vi "Read Single Measurement (Voltage).vi"(0 "VISA resource name":refnum<visa-resource-name>, 5 "Maximum Time (10000 ms)":i32=10000, 11 "error in (no error)":errorcluster) -> (4 "VISA resource name out":refnum<visa-resource-name>, 6 "DC Voltage":dbl, 8 "AC RMS Voltage":dbl, 10 "AC + DC RMS Voltage":dbl, 15 "error out":errorcluster)   [LabVIEW 2019, in "Agilent 681x Series.lvlib"]
doc: "Initiates and reads an instantaneous voltage measurement.\n\n<B>Note:</B>\n\nThis VI changes the <B>Trigger Source</B> to <B>Bus</B> and uses a software trigger after the instrument is initiated. If you want to control the triggering and other features, please use the low level VIs."
uses:
  <instrlib>/Agilent 681x Series/Agilent 681x Series.lvlib
  <instrlib>/Agilent 681x Series/Public/Data/Low Level/Fetch Single Measurement (Voltage).vi
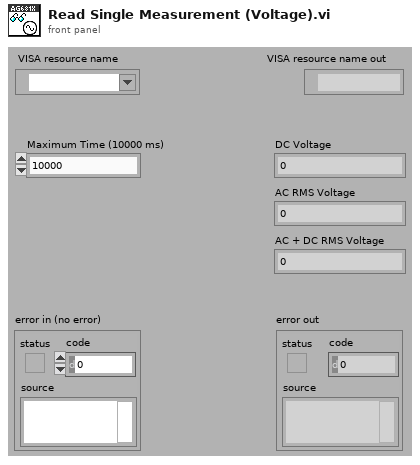
[diagram p1: front panel]
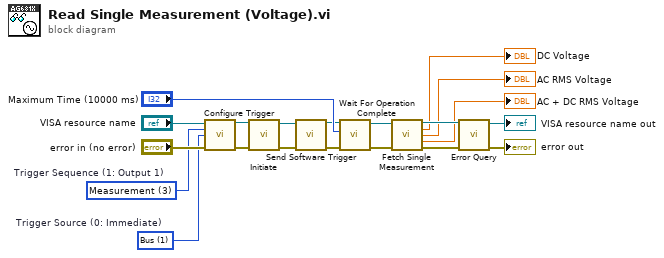
[diagram p0: block diagram]
diagram:
  w10 = 1 items=["Immediate", "Bus", "External", "Phase", "Trigger Out"]  # Trigger Source (0: Immediate)
  w11 = 3 items=["Output"=1, "Synchronous Source"=2, "Measurement"=3]  # Trigger Sequence (1: Output 1)
  n1 = call <instrlib>:"Configure Trigger.vi"("VISA resource name"="VISA resource name", "Trigger Sequence (1: Output 1)"=w11, "Trigger Source (0: Immediate)"=w10, "error in (no error)"="error in (no error)") -> ("VISA resource name out"=w8:refnum<visa-resource-name>, "error out"=w9:errorcluster)  [unwired: 10 in]
  n2 = call <instrlib>:"Initiate.vi"("error in (no error)"=w9, "VISA resource name"=w8) -> ("error out"=w7:errorcluster, "VISA resource name out"=w6:refnum<visa-resource-name>)  [unwired: 8 in]
  n3 = call <instrlib>:"Send Software Trigger.vi"("VISA resource name"=w6, "error in (no error)"=w7) -> ("VISA resource name out"=w5:refnum<visa-resource-name>, "error out"=w4:errorcluster)  [unwired: 12 in]
  n4 = call <instrlib>:"Wait For Operation Complete.vi"("error in (no error)"=w4, "Maximum Time (10000 ms)"="Maximum Time (10000 ms)", "VISA resource name"=w5) -> ("error out"=w19:errorcluster, "VISA resource name out"=w16:refnum<visa-resource-name>)  [unwired: 7 in]
  n5 = call-poly <instrlib>:"Fetch Single Measurement.vi"("VISA resource name"=w16, "error in (no error)"=w19) -> ("VISA resource name out"=w18:refnum<visa-resource-name>, "DC Voltage"=→"DC Voltage":dbl, "AC RMS Voltage"=→"AC RMS Voltage":dbl, "AC + DC RMS Voltage"=→"AC + DC RMS Voltage":dbl, "error out"=w17:errorcluster)  [unwired: 9 in]
  n6 = call <instrlib>:"Error Query.vi"("error in (no error)"=w17, "VISA resource name"=w18) -> ("error out"=→"error out":errorcluster, "VISA resource name out"=→"VISA resource name out":refnum<visa-resource-name>)  [unwired: 6 in, 2 out]
